vi "RDMA - Create Tx Transfer.vi"(0 "local address":string="169.254.239.43", 5 "local port":string, 7 "tx channels":T4[](array[typedef]) {"core"."string offset" format="%d bytes"}, 9 "destination address":string="169.254.184.119", 11 "destination port":string) -> (8 "Transfer":T1={"core"={"name"="Transfer"}, "component settings"=[], "channels"=[]} {"channels"."core"."string offset" format="%d bytes"})   [LabVIEW 2023]
uses:
  Public/Documents/National Instruments/NI VeriStand 2023/Custom Devices/Data Sharing Framework/Windows/DSF Core.lvlibp/Typedefs/DSF Engine Channel Configuration.ctl
  Public/Documents/National Instruments/NI VeriStand 2023/Custom Devices/Data Sharing Framework/Windows/DSF Core.lvlibp/Typedefs/Core Channel Configuration.ctl
  Public/Documents/National Instruments/NI VeriStand 2023/Custom Devices/Data Sharing Framework/Windows/DSF Core.lvlibp/Typedefs/DSF Data Type.ctl
  Public/Documents/National Instruments/NI VeriStand 2023/Custom Devices/Data Sharing Framework/Windows/DSF Core.lvlibp/Typedefs/DSF Settings Info.ctl
  Public/Documents/National Instruments/NI VeriStand 2023/Custom Devices/Data Sharing Framework/Windows/DSF Core.lvlibp/Typedefs/DSF Engine Transfer Configuration.ctl
  Public/Documents/National Instruments/NI VeriStand 2023/Custom Devices/Data Sharing Framework/Windows/DSF Core.lvlibp/Typedefs/Core Transfer Configuration.ctl
  Public/Documents/National Instruments/NI VeriStand 2023/Custom Devices/Data Sharing Framework/Windows/DSF Core.lvlibp
  Public/Documents/National Instruments/NI VeriStand 2023/Custom Devices/Data Sharing Framework/Windows/DSF Core.lvlibp/Classes/Configuration/Core/Channel/Channel Configuration.lvclass
  Public/Documents/National Instruments/NI VeriStand 2023/Custom Devices/Data Sharing Framework/Windows/DSF Core.lvlibp/Classes/Configuration/Core/Transfer/Transfer Configuration.lvclass
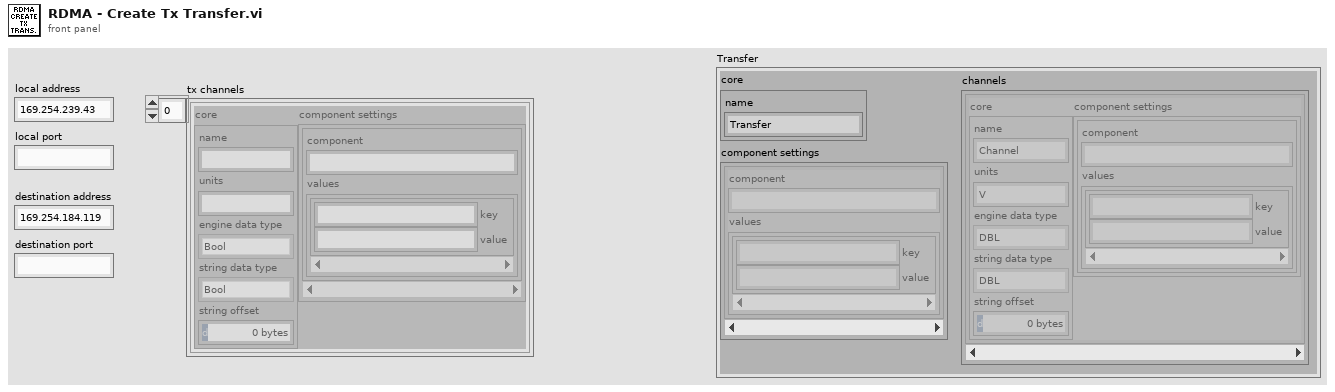
[diagram p1: front panel]
types:
  T1 = typedef "DSF Core.lvlibp/DSF Engine Transfer Configuration.ctl" = cluster{"core":T2, "component settings":T3[], "channels":T4[]}
  T2 = typedef "DSF Core.lvlibp/Transfer Configuration.lvclass/Core Transfer Configuration.ctl" = cluster{"name":string}
  T3 = typedef "DSF Core.lvlibp/DSF Settings Info.ctl" = cluster{"component":string, "values":cluster{"key":string, "value":string}[]}
  T4 = typedef "DSF Core.lvlibp/DSF Engine Channel Configuration.ctl" = cluster{"core":T5, "component settings":T3[]}
  T5 = typedef "DSF Core.lvlibp/Channel Configuration.lvclass/Core Channel Configuration.ctl" = cluster{"name":string, "units":string, "engine data type":T6, "string data type":T6, "string offset":u64}
  T6 = typedef "DSF Core.lvlibp/DSF Data Type.ctl" = enum8{"Bool", "SGL", "DBL", "I8", "I16", "I32", "I64", "U8", "U16", "U32", "U64"}
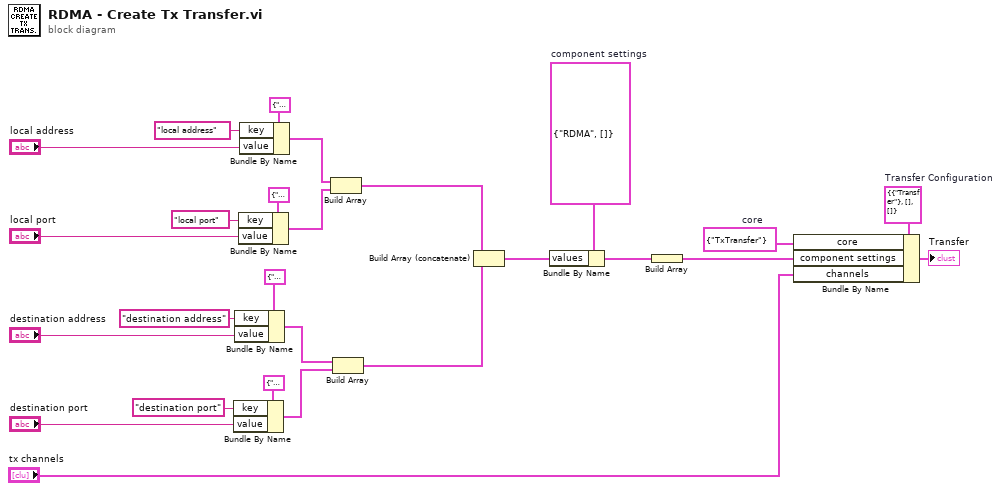
[diagram p0: block diagram]
diagram:
  w24 = T3 {"component"="RDMA", "values"=[]}  # component settings
  w25 = T2 {"name"="TxTransfer"}  # core
  w26 = T1 {"core"={"name"="Transfer"}, "component settings"=[], "channels"=[]}  # Transfer Configuration
  n1 = Bundle By Name(cluster=cluster{"key":string, "value":string} {"key"="", "value"=""} ("setting"), "key"="destination port", "value"="destination port") -> (w12:cluster{"key":string, "value":string})
  n2 = Bundle By Name(cluster=cluster{"key":string, "value":string} {"key"="", "value"=""} ("setting"), "key"="destination address", "value"="destination address") -> (w13:cluster{"key":string, "value":string})
  n3 = Bundle By Name(cluster=cluster{"key":string, "value":string} {"key"="", "value"=""} ("setting"), "key"="local port", "value"="local port") -> (w6:cluster{"key":string, "value":string})
  n4 = Bundle By Name(cluster=cluster{"key":string, "value":string} {"key"="", "value"=""} ("setting"), "key"="local address", "value"="local address") -> (w9:cluster{"key":string, "value":string})
  n5 = Build Array(w9, w6) -> (w3:cluster{"key":string, "value":string}[])
  n6 = Build Array(w13, w12) -> (w5:cluster{"key":string, "value":string}[])
  n7 = Build Array (concatenate)(w3, w5) -> (w4:cluster{"key":string, "value":string}[])
  n8 = Bundle By Name(cluster=w24, "values"=w4) -> (w10:T3)
  n9 = Build Array(w10) -> (w11:T3[])
  n10 = Bundle By Name(cluster=w26, "core"=w25, "component settings"=w11, "channels"="tx channels") -> (→"Transfer":T1)
